vi "resetForceActuators.vi"(8 "error in (no error)":errorcluster, 11 "Model in":refnum<class "Model.lvclass">) -> (0 "error out":errorcluster, 3 "Model out":refnum<class "Model.lvclass">)   [LabVIEW 2016, in "Model.lvclass"]
uses:
  Model.lvclass
  Model.lvclass/Model.ctl
  ILCCommunications/ILCCommunications.lvclass/ILCCommunications.ctl
  Common_RT_ILC/ILC/ILC.lvclass/ILC.ctl
  Common_RT_Modbus/ModbusBuffer/ModbusBuffer.lvclass/ModbusBuffer.ctl
  ILCCommunications/resetFA.vi
  ILCCommunications/reset.vi
  Common_RT_ILC/ILC/addResetFrame.vi
  Common_RT_Modbus/ModbusBuffer/writeHeader.vi
  Common_RT_Modbus/ModbusBuffer/writeU8.vi
  Common_RT_Modbus/ModbusBuffer/writeCRC.vi
  Common_RT_Modbus/ModbusBuffer/writeEndOfFrame.vi
  Common_RT_Modbus/ModbusBuffer/writeWaitForRx.vi
  Common_RT_Modbus/ModbusBuffer/writeByteInstruction.vi
  Common_RT_Modbus/ModbusBuffer/calculateCRC.vi
  Common_RT_FAILC/FAILC/FAILC.lvclass
  D:/Code/ts_M1M3Support/Common_RT_ILC/ILC/ILC.lvclass
  ILCCommunications/ILCCommunications.lvclass
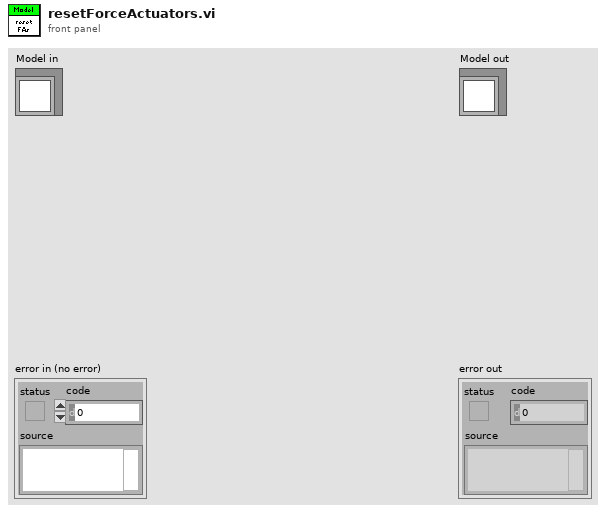
[diagram p1: front panel]
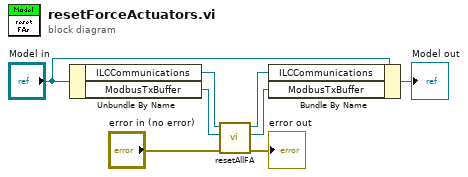
[diagram p0: block diagram]
diagram:
  n1 = Unbundle By Name("Model in") -> ("ILCCommunications"=w6:refnum<class "ILCCommunications.lvclass">, "ModbusTxBuffer"=w5:refnum<class "ModbusBuffer.lvclass">)
  n2 = call "resetAllFA.vi"("error in (no error)"="error in (no error)", "ModbusBuffer in"=w5, "ILCCommunications in"=w6) -> ("error out"=→"error out":errorcluster, "ModbusBuffer out"=w2:refnum<class "ModbusBuffer.lvclass">, "ILCCommunications out"=w1:refnum<class "ILCCommunications.lvclass">)  [unwired: 6 in]
  n3 = Bundle By Name(cluster="Model in", "ILCCommunications"=w1, "ModbusTxBuffer"=w2) -> (→"Model out":refnum<class "Model.lvclass">)
